vi "signal_gen.vi"() -> ()   [LabVIEW 2013]
panel:
  in  "+szum":bool
  in  "+square":bool
  out "suma":dynamicdata(graph)
  in  "Offset sqaure":dbl caption="Offset"
  in  "odchylenie std. szum":dbl=0.6 caption="Standard deviation"
  in  "Phase szum":dbl caption="Phase"
  in  "Amplitude szum":dbl=1.0 caption="Amplitude"
  in  "Frequency szum":dbl=10.1 caption="Frequency"
  in  "Offset szum":dbl caption="Offset"
  in  "Phase sin":dbl caption="Phase"
  in  "Amplitude sin":dbl=1.0 caption="Amplitude"
  in  "Frequency sin":dbl=10.1 caption="Frequency"
  in  "Offset sin":dbl caption="Offset"
  in  "Phase square":dbl caption="Phase"
  in  "amp. square":dbl=1.0 caption="Amplitude"
  in  "freq. square":dbl=10.1 caption="Frequency"
  in  "stop":bool
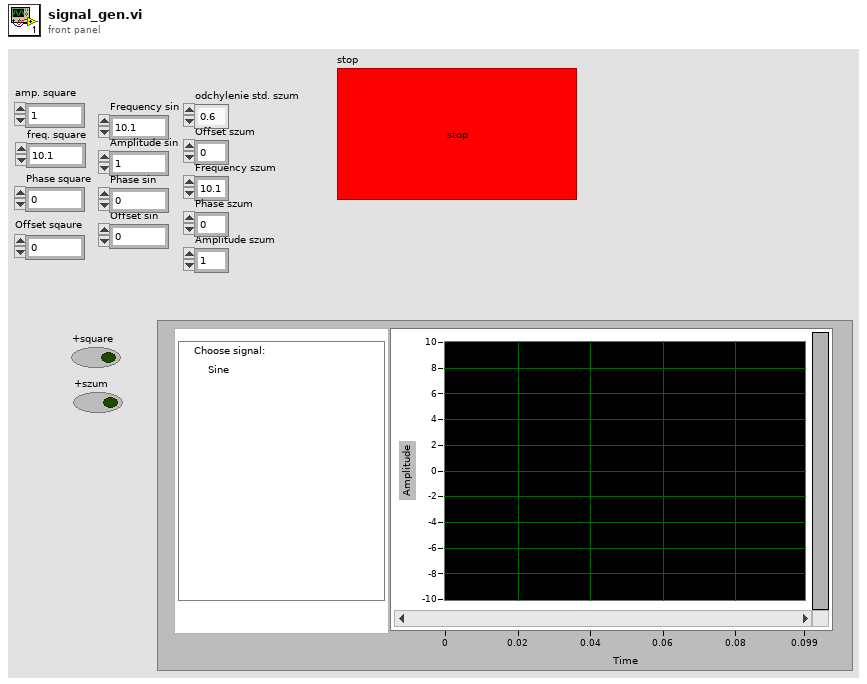
[diagram p1: front panel]
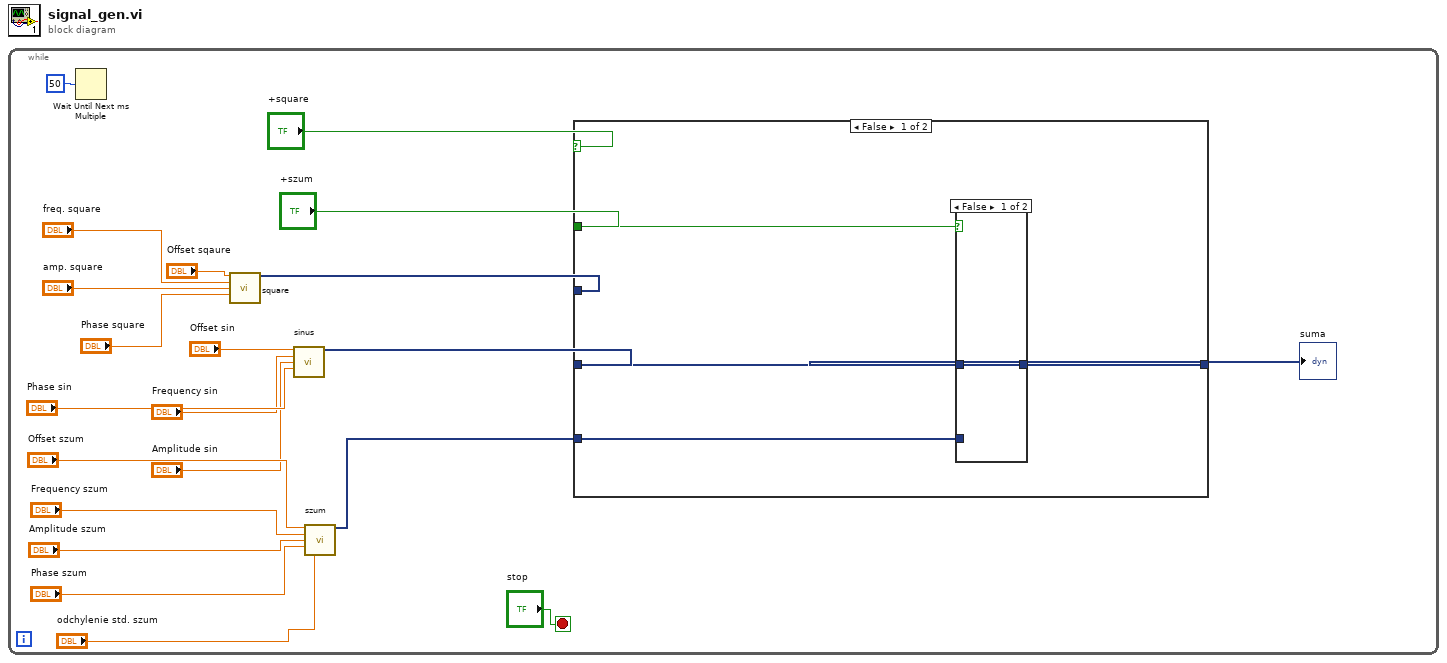
[diagram p0: block diagram]
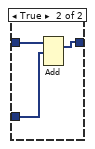
[diagram p2: hidden frame]
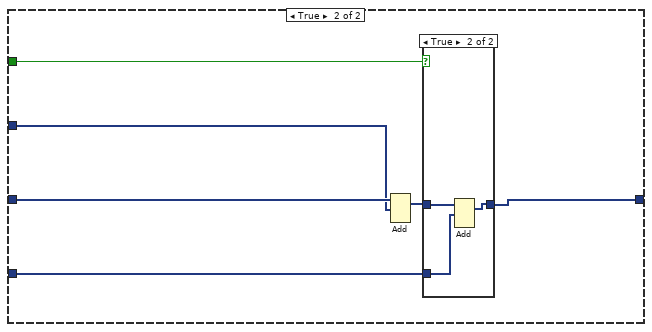
[diagram p3: hidden frame]
diagram:
  n1 = while {
    stop <- "stop" stop-if-true
    n2 = Wait Until Next ms Multiple(millisecond multiple=u32 50) -> ()  [unwired: 1 out]
    n3 = call "square"("Offset"="Offset sqaure", "Frequency"="freq. square", "Amplitude"="amp. square", "Phase"="Phase square") -> ("Square"=w5:dynamicdata)  [unwired: 10 in, 1 out]
    n4 = call "sinus"("Offset"="Offset sin", "Frequency"="Frequency sin", "Amplitude"="Amplitude sin", "Phase"="Phase sin") -> ("Sine"=w6:dynamicdata)  [unwired: 10 in, 1 out]
    n5 = call "szum"("Offset"="Offset szum", "Frequency"="Frequency szum", "Amplitude"="Amplitude szum", "Phase"="Phase szum", "Standard deviation"="odchylenie std. szum") -> ("Sine with Gaussian Noise"=w2:dynamicdata)  [unwired: 9 in, 1 out]
    n6 = case shown="False" "+square" {
      tunnel: w6 -> [w24 w35]
      tunnel: w5 -> [_ w34]
      tunnel: "+szum" -> [w25 w32]
      tunnel: w2 -> [w23 w31]
      tunnel: [w22 w30] -> w1
      frame False {
        n7 = case shown="False" w25 {
          tunnel: w24 -> [w26 w29]
          tunnel: w23 -> [_ w28]
          tunnel: [w26 w27] -> w22
          frame False {
          }
          frame True {
            n8 = Add(1:w28, 2:w29) -> (0:w27:dynamicdata)  [unwired: 1 in, 1 out]
          }
        }
      }
      frame True {
        n9 = Add(1:w34, 2:w35) -> (0:w33:dynamicdata)  [unwired: 1 in, 1 out]
        n10 = case shown="True" w32 {
          tunnel: w33 -> [w36 w39]
          tunnel: w31 -> [_ w38]
          tunnel: [w36 w37] -> w30
          frame False {
          }
          frame True {
            n11 = Add(1:w38, 2:w39) -> (0:w37:dynamicdata)  [unwired: 1 in, 1 out]
          }
        }
      }
    }
    "suma" <- w1
  }
